vi "sync start of cycle.vi"(8 "error in (no error)":errorcluster, 11 "module in":refnum<class "Shared Memory runtime.lvclass">) -> (0 "error out":errorcluster, 3 "module out":refnum<class "Shared Memory runtime.lvclass">)   [LabVIEW 2013, in "Shared Memory runtime.lvclass"]
uses:
  Shared Memory runtime.lvclass
  Shared Memory runtime.lvclass/Shared Memory runtime.ctl
  Read sync data.vi
  <vilib>/NI/Pthreads for LabVIEW on Linux RT/Classes/Semaphore/Semaphore.lvclass
  <vilib>/NI/Shared Memory Library/Classes/Shared Memory/Shared Memory.lvclass
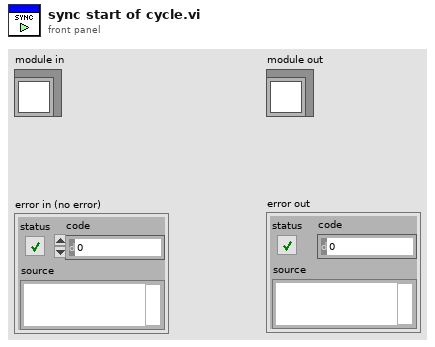
[diagram p1: front panel]
types:
  T1 = typedef "Shared Memory runtime.lvclass/sync data.ctl" = cluster{"semaphores soc":T2[], "semaphores eoc":T2[], "timeout":dbl, "enabled":bool, "sync shared memory":T4}
  T2 = typedef "Shared Memory runtime.lvclass/semaphore data.ctl" = cluster{"semaphore":T3, "name":string}
  T3 = typedef "POSIX Threads.lvlib/Semaphore.lvclass/reference.ctl" = refnum<data-value>
  T4 = typedef "Shared Memory.lvlib/Shared Memory.lvclass/reference.ctl" = refnum<data-value>
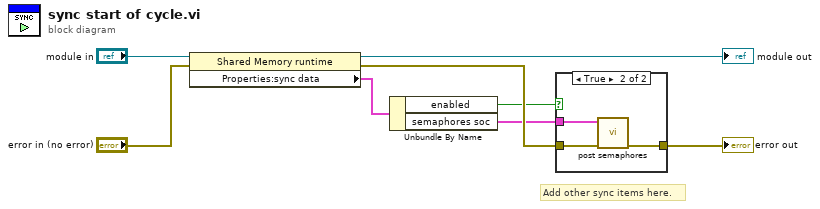
[diagram p0: block diagram]
diagram:
  # "Add other sync items here."
  n1 = property class="Shared Memory runtime"(reference="module in", error in="error in (no error)") -> (reference out=→"module out":refnum<class "Shared Memory runtime.lvclass">, error out=w4:errorcluster, "Properties:sync data"=w5:T1)
  n2 = Unbundle By Name(w5) -> ("enabled"=w1:bool, "semaphores soc"=w3:T2[])
  n3 = case shown="True" w1 {
    tunnel: w4 -> [w9 w12]
    tunnel: w3 -> [_ w11]
    tunnel: [w9 w10] -> w2
    frame False {
    }
    frame True {
      n4 = call "post semaphores.vi"("error in (no error)"=w12, "semaphores in"=w11) -> ("error out"=w10:errorcluster)  [unwired: 8 in, 1 out]
    }
  }
  "error out" <- w2
